vi "Constants.vi"() -> ()   [LabVIEW 2019, in "VCD Debug Tools Dependencies.lvlib"]
uses:
  HLA Custom Device Configuration.llb/VCD Debug Tools Dependencies.lvlib
panel:
  in  "Status String Format String":string="%%LABEL%%%s%%LABEL%%\n%%STATUS%%%s%%STATUS%%"
  in  "Transmit Overflow Tag":string="##TRANSMIT BUFFER OVERFLOW##"
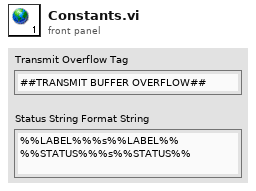
[diagram p1: front panel]
diagram:
